vi "Warn Deprecated VI.vi"(8 "error in (no error)":errorcluster, 9 "replacement":string, 10 "deprecated version":string) -> (0 "error out":errorcluster)   [LabVIEW 2017, in "libssh2.lvlib"]
uses:
  libssh2.lvlib
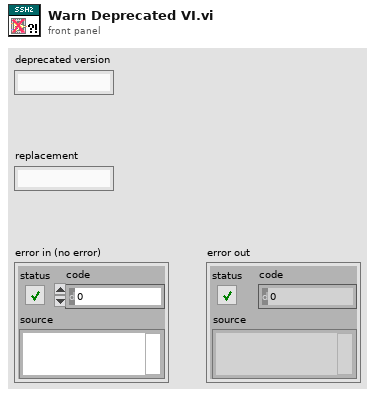
[diagram p1: front panel]
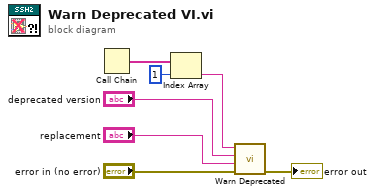
[diagram p0: block diagram]
diagram:
  n1 = Call Chain() -> (call chain=w7:string[])
  n2 = Index Array(array=w7, index=1) -> (element=w1:string)
  n3 = call "Warn Deprecated.vi"("error in (no error)"="error in (no error)", "replacement"="replacement", "deprecated version"="deprecated version", "name"=w1) -> ("error out"=→"error out":errorcluster)  [unwired: 7 in]
